vi "OldIntakeExecuteLogic.vi"(9 "HaveNoteSensor":bool, 11 "Sensor Velocity":dbl) -> (1 "MotorOutDmd 2":dbl, 3 "MotorOutDmd":dbl)   [LabVIEW 2023]
uses:
  OldIntakeState.ctl
  <vilib>/Rock Robotics/WPI/ThirdParty/JAS_Junk/TrajLib/VI/BoolCmd_Recv_Internal.vi
  <vilib>/Rock Robotics/WPI/ThirdParty/JAS_Junk/TrajLib/VI/DigSeqLogic_Edge_On.vi
  <vilib>/Rock Robotics/WPI/ThirdParty/JAS_Junk/TrajLib/VI/BoolCmd_ObtainQueue.vi
  OldIntakeGlobal.vi
  <vilib>/Rock Robotics/WPI/ThirdParty/JAS_Junk/TrajLib/Trajectory_Library.lvlib
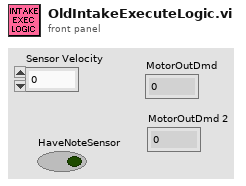
[diagram p1: front panel]
types:
  T1 = typedef "OldIntakeState.ctl" = enum16{"0-init", "1-cancel", "2-wait-for-cmd", "3-intake-check-for-note", "4-intake-start-intake", "5-intake-have-note-yet", "6-intake-stop-motor", "7-spit-out", "8-feed-note-to-shooter"}
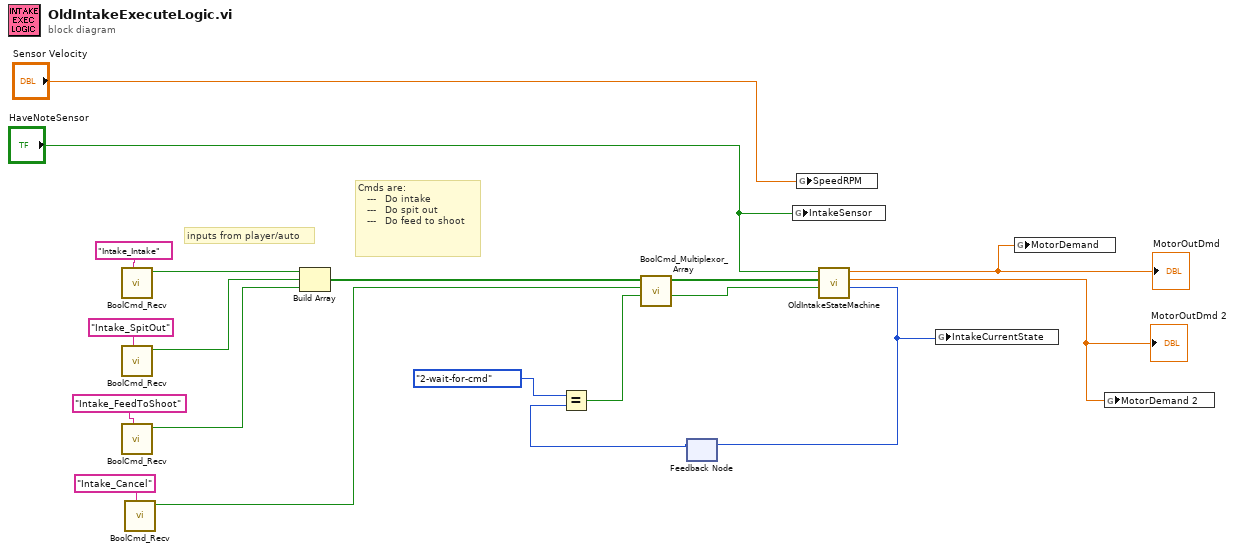
[diagram p0: block diagram]
diagram:
  # "Cmds are:\n   ---   Do intake\n   ---   Do spit out\n   ---   Do feed to shoot"
  # "inputs from player/auto"
  n1 = call <vilib>:"BoolCmd_Recv.vi"("Command Name"="Intake_Intake") -> ("New Request"=w7:bool)  [unwired: 9 in, 1 out]
  n2 = call <vilib>:"BoolCmd_Recv.vi"("Command Name"="Intake_SpitOut") -> ("New Request"=w6:bool)  [unwired: 9 in, 1 out]
  n3 = call <vilib>:"BoolCmd_Recv.vi"("Command Name"="Intake_FeedToShoot") -> ("New Request"=w4:bool)  [unwired: 9 in, 1 out]
  n4 = call <vilib>:"BoolCmd_Recv.vi"("Command Name"="Intake_Cancel") -> ("New Request"=w9:bool)  [unwired: 9 in, 1 out]
  n5 = Build Array(w7, w6, w4) -> (w8:bool[])
  n6 = feedback #1() -> (w16:T1)  [unwired: 1 in]
  n7 = Equal?(x=OldIntakeState."2-wait-for-cmd", y=w16) -> (x = y?=w15:bool)
  n8 = call <vilib>:"BoolCmd_Multiplexor_Array.vi"("Ready"=w15, "Command Cancel"=w9, "Commands"=w8) -> ("Do Cancel"=w14:bool, "Do Command"=w13:bool[])  [unwired: 7 in]
  n9 = global write "OldIntakeGlobal.vi" "IntakeSensor"("HaveNoteSensor") -> ()
  n10 = global write "OldIntakeGlobal.vi" "SpeedRPM"("Sensor Velocity") -> ()
  n11 = call "OldIntakeStateMachine.vi"("IntakeCancel"=w14, "IntakeCommand"=w13, "Sensor_HaveNote"="HaveNoteSensor") -> ("Intake_State"=w2:T1, "MotorOutDmd 2"=w1:dbl, "MotorOutDmd"=w3:dbl)  [unwired: 5 in, 1 out]
  "MotorOutDmd" <- w3
  "MotorOutDmd 2" <- w1
  n12 = feedback-in #1(w2) -> ()
  n13 = global write "OldIntakeGlobal.vi" "IntakeCurrentState"(w2) -> ()
  n14 = global write "OldIntakeGlobal.vi" "MotorDemand"(w3) -> ()
  n15 = global write "OldIntakeGlobal.vi" "MotorDemand 2"(w1) -> ()
